vi "Thorlabs-Update Settings.vi"(8 "error in (no error)":errorcluster, 10 "params":variant=variant(cluster{"New LSM Settings":cluster{"Multi Frame Count":dbl, "Trigger Mode":dbl, "Channel Selection":enum32{"A", "B", "AB"}, "Pixel Count":cluster{"Pixels in X":u32, "Pixels in Y":u32}, "Field Size":dbl, "Area Mode":dbl, "Frames":u8, "Averaging":bool, "Alignment":dbl, "Scan Mode":bool, "Gain":cluster{"Gain A":u8, "Gain B":u8}, "Enable PMTs":cluster{"A":bool, "B":bool}, "Voltage Range":cluster{"Range A":u16, "Range B":u16}, "Real Time Averaging":bool, "PFOV":dbl, "MicronsPerPx":dbl}, "index of element":i32} {"New LSM Settings"={"Multi Frame Count"=0.0, "Trigger Mode"=2.0, "Channel Selection"=enum."A", "Pixel Count"={"Pixels in X"=32, "Pixels in Y"=32}, "Field Size"=90.0, "Area Mode"=1.0, "Frames"=2, "Averaging"=FALSE, "Alignment"=0.0, "Scan Mode"=TRUE, "Gain"={"Gain A"=1, "Gain B"=1}, "Enable PMTs"={"A"=TRUE, "B"=TRUE}, "Voltage Range"={"Range A"=10, "Range B"=10}, "Real Time Averaging"=TRUE, "PFOV"=0.0, "MicronsPerPx"=0.0}, "index of element"=13})) -> (0 "error out":errorcluster, 2 "Pause Live Imaging":bool)   [LabVIEW 2020]
uses:
  _Controls/Confocal Controls.ctl
  _Globals/Global Controls.vi
  _Globals/pDataBuffer.vi
  LSM_SDK/ThorConfocal.lvlib
  ECU_SDK/ThorECU.lvlib
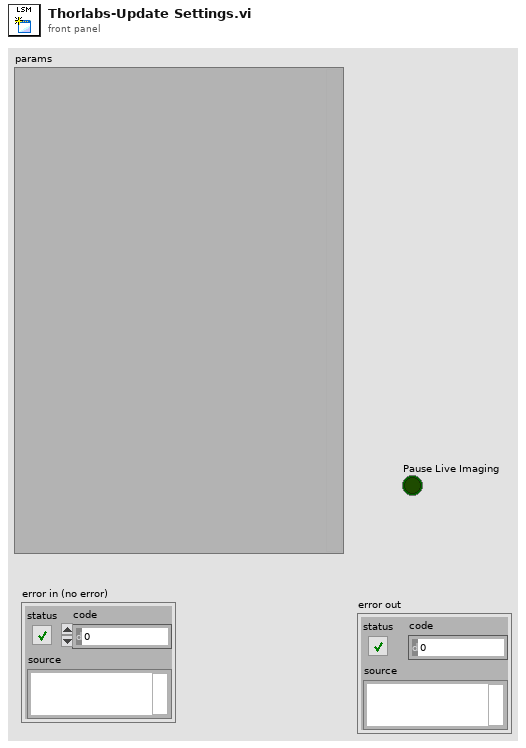
[diagram p1: front panel]
types:
  T1 = typedef "Confocal Controls.ctl" = cluster{"Channel Selection":enum32{"A", "B", "AB"}, "Pixel Count":cluster{"Pixels in X":u32, "Pixels in Y":u32}, "Field Size":dbl, "Frames":u8, "Averaging":bool, "Alignment":dbl, "Scan Mode":bool, "Gain":cluster{"Gain A":u8, "Gain B":u8}, "Enable PMTs":cluster{"A":bool, "B":bool}, "Voltage Range":cluster{"Range A":u16, "Range B":u16}, "Multi Frame Count":dbl, "Trigger Mode":dbl, "Real Time Averaging":bool, "PFOV":dbl, "MicronsPerPx":dbl}
  T2 = cluster{"Newest LSM Settings":T1, "Index of Change":i32}
  T3 = typedef "Tweezertron Ctrl Refs.ctl" = cluster{"LSM Settings":refnum<vi>, "iFlex Control":refnum<vi>, "PIFOC Settings":refnum<vi>, "PinSelector":refnum<vi>, "Manlight Controls":refnum<vi>, "Exp Params":refnum<vi>, "Image Thresholds":refnum<vi>}
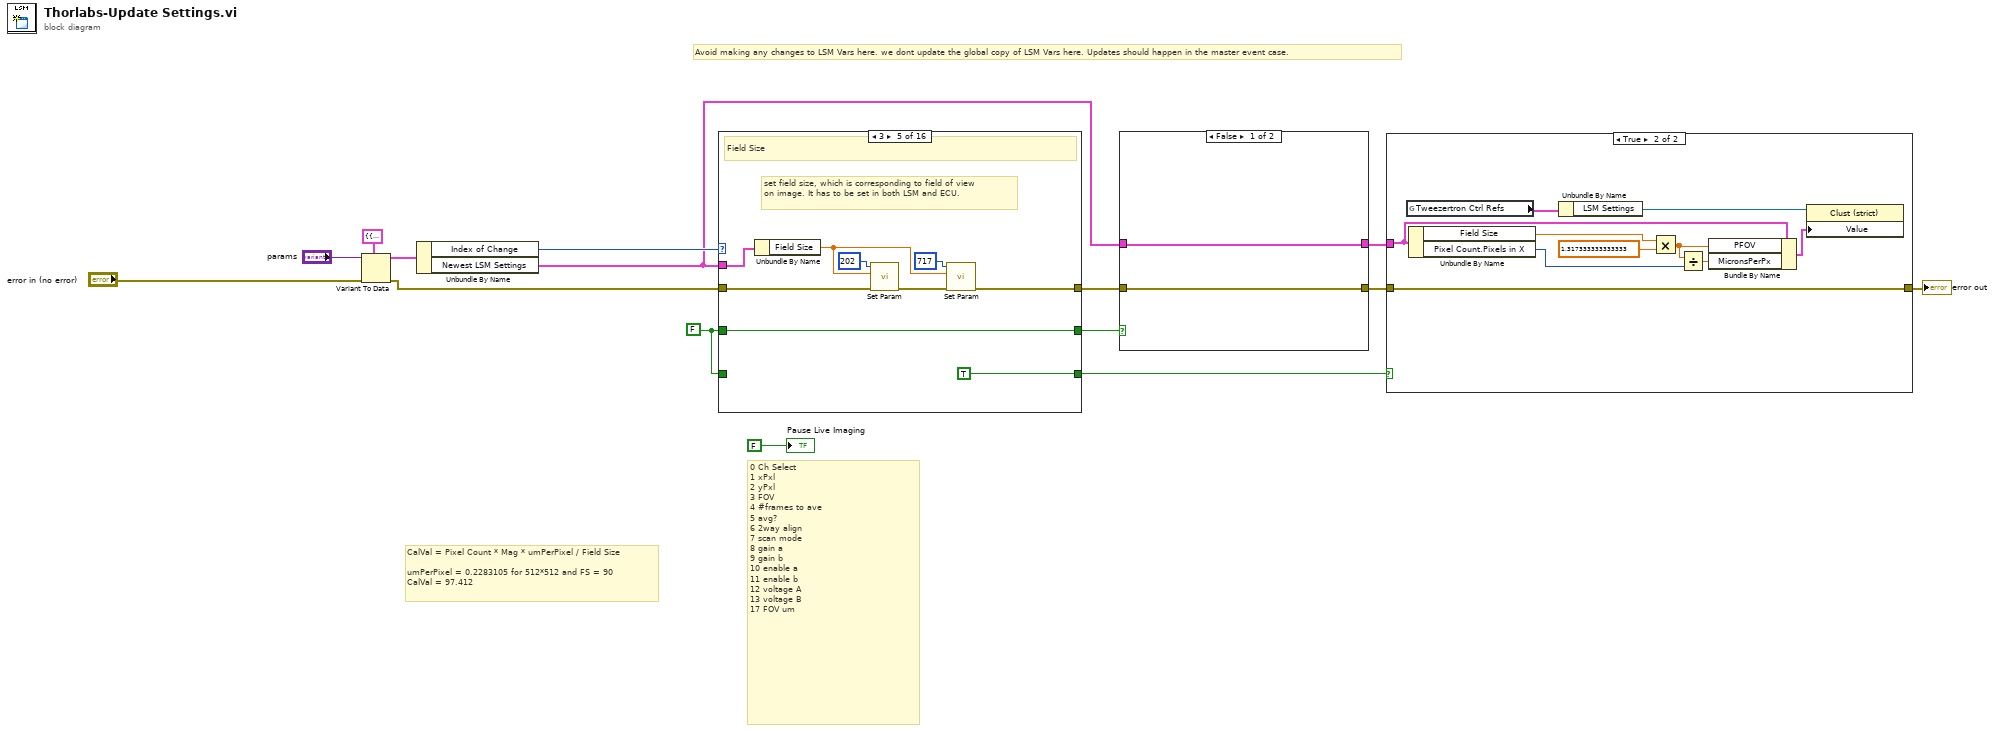
[diagram p0: block diagram]
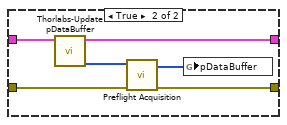
[diagram p3: hidden frame]
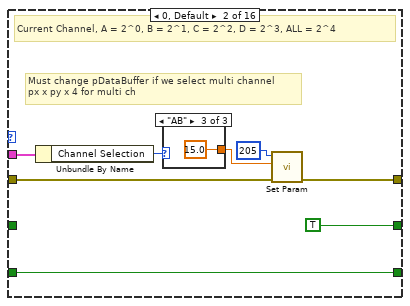
[diagram p5: hidden frame]
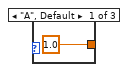
[diagram p6: hidden frame]
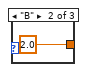
[diagram p7: hidden frame]
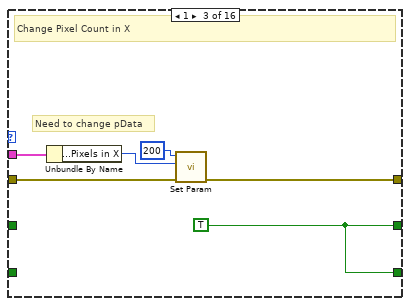
[diagram p8: hidden frame]
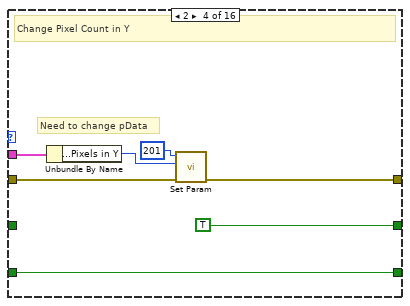
[diagram p9: hidden frame]
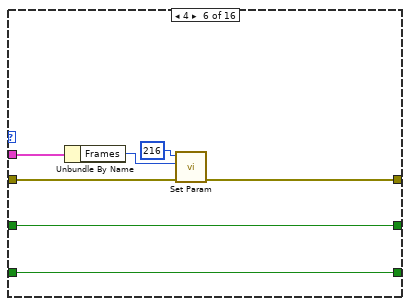
[diagram p10: hidden frame]
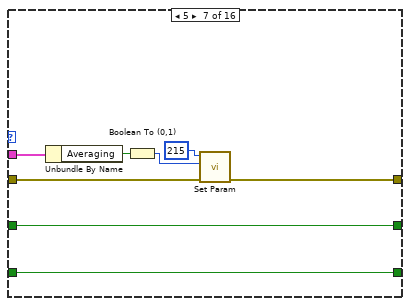
[diagram p11: hidden frame]
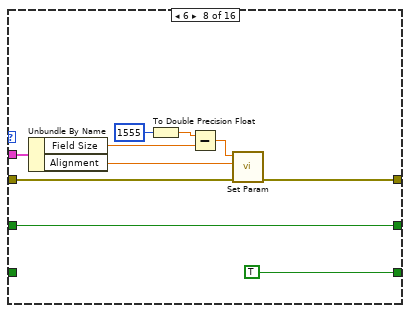
[diagram p12: hidden frame]
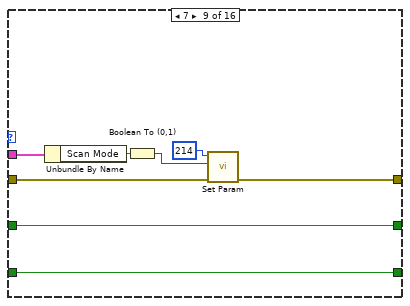
[diagram p13: hidden frame]
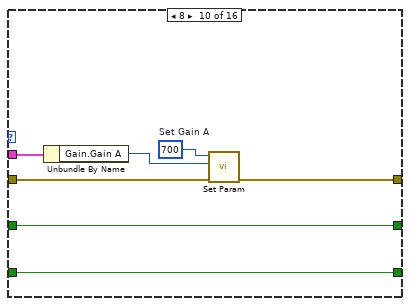
[diagram p14: hidden frame]
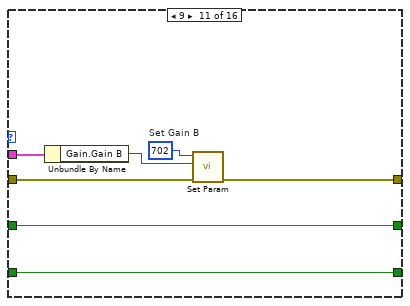
[diagram p15: hidden frame]
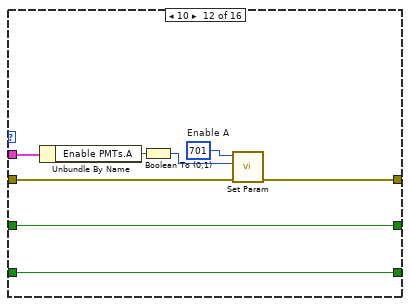
[diagram p16: hidden frame]
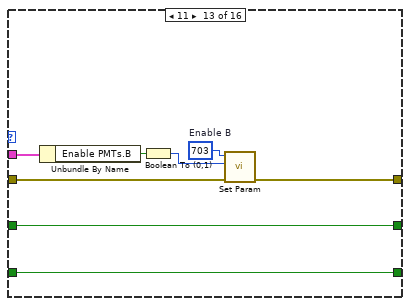
[diagram p17: hidden frame]
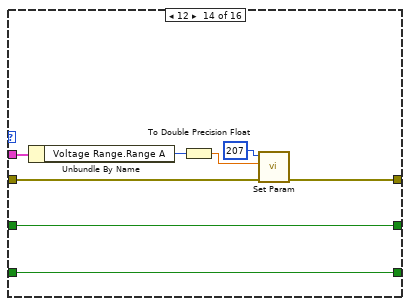
[diagram p18: hidden frame]
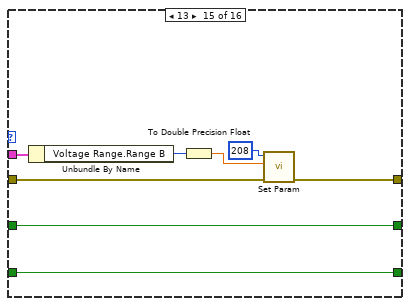
[diagram p19: hidden frame]
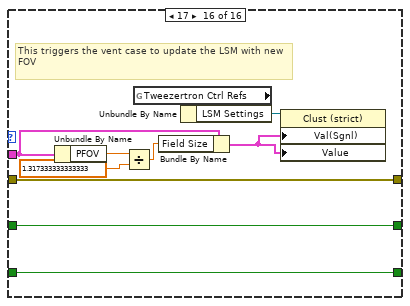
[diagram p20: hidden frame]
diagram:
  w5 = FALSE
  # "Avoid making any changes to LSM Vars here. we dont update the global copy of LSM Vars here. Updates should happen in the master event case."
  # "CalVal = Pixel Count * Mag * umPerPixel / Field Size\n\numPerPixel = 0.2283105 for 512*512 and FS = 90\nCalVal = 97.412"
  # "0 Ch Select \n1 xPxl\n2 yPxl\n3 FOV\n4 #frames to ave\n5 avg?\n6 2way align\n7 scan mode\n8 gain a\n9 gain b\n10 enable a\n11 enable b\n12 voltage A\n13 voltage B\n17 FOV um"
  n1 = Variant To Data(error in="error in (no error)", type=T2 {"Newest LSM Settings"={"Channel Selection"=enum."A", "Pixel Count"={"Pixels in X"=512, "Pixels in Y"=512}, "Field Size"=30.0, "Frames"=0, "Averaging"=FALSE, "Alignment"=0.0, "Scan Mode"=TRUE, "Gain"={"Gain A"=0, "Gain B"=0}, "Enable PMTs"={"A"=FALSE, "B"=FALSE}, "Voltage Range"={"Range A"=10, "Range B"=7}, "Multi Frame Count"=0.0, "Trigger Mode"=2.0, "Real Time Averaging"=TRUE, "PFOV"=0.0, "MicronsPerPx"=0.0}, "Index of Change"=0} ("output cluster"), Variant="params") -> (data=w13:T2, error out=w11:errorcluster)
  n2 = Unbundle By Name(w13) -> ("Index of Change"=w15:i32, "Newest LSM Settings"=w6:T1)
  n3 = case shown="3" w15 {
    tunnel: w6 -> [_ w23 w32 w39 w46 w56 w63 w74 w82 w90 w94 w104 w109 w117 w128 w134]
    tunnel: w11 -> [w18 w25 w35 w42 w51 w58 w66 w76 w84 w88 w96 w106 w111 w122 w129 w133]
    tunnel: [w18 w24 w34 w41 w49 w54 w65 w75 w79 w87 w95 w105 w110 w121 w127 w133] -> w7
    tunnel: [w17 TRUE w30 TRUE w44 w53 w60 w68 w78 w86 w93 w100 w108 w116 w124 w140] -> w8
    tunnel: w5 -> [w17 _ _ _ w44 w53 w60 w68 w78 w86 w93 w100 w108 w116 w124 w140]
    tunnel: w5 -> [w16 w19 _ w36 _ w52 w59 _ w77 w85 w92 w99 w107 w115 w123 w132]
    tunnel: [w16 w19 w30 w36 TRUE w52 w59 TRUE w77 w85 w92 w99 w107 w115 w123 w132] -> w4
    frame -1 {
      # "If nothing changed, do nothing"
    }
    frame 0, Default {
      # "Must change pDataBuffer if we select multi channel\npx x py x 4 for multi ch"
      # "Current Channel, A = 2^0, B = 2^1, C = 2^2, D = 2^3, ALL = 2^4"
      n4 = Unbundle By Name(w23) -> ("Channel Selection"=w22:enum32{"A", "B", "AB"})
      n5 = case shown="\"AB\"" w22 {
        tunnel: [1.0 ("f") 2.0 15.0] -> w21
        frame "A", Default {
        }
        frame "B" {
        }
        frame "AB" {
        }
      }
      n6 = call "Set Param.vi"("error in (no error)"=w25, "param"=w21, "paramID"=205) -> ("error out"=w24:errorcluster)  [unwired: 3 in, 1 out]
    }
    frame 1 {
      w30 = TRUE
      # "Need to change pData"
      # "Change Pixel Count in X"
      n7 = Unbundle By Name(w32) -> ("Pixel Count.Pixels in X"=w31:u32)
      n8 = call "Set Param.vi"("error in (no error)"=w35, "param"=w31, "paramID"=200) -> ("error out"=w34:errorcluster)  [unwired: 3 in, 1 out]
    }
    frame 2 {
      # "Need to change pData"
      # "Change Pixel Count in Y"
      n9 = Unbundle By Name(w39) -> ("Pixel Count.Pixels in Y"=w38:u32)
      n10 = call "Set Param.vi"("error in (no error)"=w42, "param"=w38, "paramID"=201) -> ("error out"=w41:errorcluster)  [unwired: 3 in, 1 out]
    }
    frame 3 {
      # "set field size, which is corresponding to field of view \non image. It has to be set in both LSM and ECU."
      # "Field Size"
      n11 = Unbundle By Name(w46) -> ("Field Size"=w45:dbl)
      n12 = call "Set Param.vi"("error in (no error)"=w51, "param"=w45, "paramID"=202) -> ("error out"=w50:errorcluster)  [unwired: 3 in, 1 out]
      n13 = call "Set Param.vi"("error in (no error)"=w50, "param"=w45, "paramID"=717) -> ("error out"=w49:errorcluster)  [unwired: 7 in, 1 out]
    }
    frame 4 {
      n14 = Unbundle By Name(w56) -> ("Frames"=w55:u8)
      n15 = call "Set Param.vi"("error in (no error)"=w58, "param"=w55, "paramID"=216) -> ("error out"=w54:errorcluster)  [unwired: 3 in, 1 out]
    }
    frame 5 {
      n16 = Unbundle By Name(w63) -> ("Averaging"=w62:bool)
      n17 = Boolean To (0,1)(Boolean=w62) -> (0, 1=w61:i16)
      n18 = call "Set Param.vi"("error in (no error)"=w66, "param"=w61, "paramID"=215) -> ("error out"=w65:errorcluster)  [unwired: 3 in, 1 out]
    }
    frame 6 {
      n19 = Unbundle By Name(w74) -> ("Field Size"=w71:dbl, "Alignment"=w73:dbl)
      n20 = To Double Precision Float(number=1555 ("paramID")) -> (double precision float=w69:dbl)
      n21 = Subtract(x=w69, y=w71) -> (x-y=w70:dbl)
      n22 = call "Set Param.vi"("error in (no error)"=w76, "param"=w73, "paramID"=w70) -> ("error out"=w75:errorcluster)  [unwired: 7 in, 1 out]
    }
    frame 7 {
      n23 = Unbundle By Name(w82) -> ("Scan Mode"=w81:bool)
      n24 = Boolean To (0,1)(Boolean=w81) -> (0, 1=w80:i16)
      n25 = call "Set Param.vi"("error in (no error)"=w84, "param"=w80, "paramID"=214) -> ("error out"=w79:errorcluster)  [unwired: 3 in, 1 out]
    }
    frame 8 {
      w91 = 700  # Set Gain A
      n26 = Unbundle By Name(w90) -> ("Gain.Gain A"=w89:u8)
      n27 = call "Set Param.vi"("error in (no error)"=w88, "param"=w89, "paramID"=w91) -> ("error out"=w87:errorcluster)  [unwired: 7 in, 1 out]
    }
    frame 9 {
      w97 = 702  # Set Gain B
      n28 = Unbundle By Name(w94) -> ("Gain.Gain B"=w98:u8)
      n29 = call "Set Param.vi"("error in (no error)"=w96, "param"=w98, "paramID"=w97) -> ("error out"=w95:errorcluster)  [unwired: 7 in, 1 out]
    }
    frame 10 {
      w102 = 701  # Enable A
      n30 = Unbundle By Name(w104) -> ("Enable PMTs.A"=w103:bool)
      n31 = Boolean To (0,1)(Boolean=w103) -> (0, 1=w101:i16)
      n32 = call "Set Param.vi"("error in (no error)"=w106, "param"=w101, "paramID"=w102) -> ("error out"=w105:errorcluster)  [unwired: 7 in, 1 out]
    }
    frame 11 {
      w112 = 703  # Enable B
      n33 = Unbundle By Name(w109) -> ("Enable PMTs.B"=w113:bool)
      n34 = Boolean To (0,1)(Boolean=w113) -> (0, 1=w114:i16)
      n35 = call "Set Param.vi"("error in (no error)"=w111, "param"=w114, "paramID"=w112) -> ("error out"=w110:errorcluster)  [unwired: 7 in, 1 out]
    }
    frame 12 {
      n36 = Unbundle By Name(w117) -> ("Voltage Range.Range A"=w119:u16)
      n37 = To Double Precision Float(number=w119) -> (double precision float=w118:dbl)
      n38 = call "Set Param.vi"("error in (no error)"=w122, "param"=w118, "paramID"=207) -> ("error out"=w121:errorcluster)  [unwired: 3 in, 1 out]
    }
    frame 13 {
      n39 = Unbundle By Name(w128) -> ("Voltage Range.Range B"=w126:u16)
      n40 = To Double Precision Float(number=w126) -> (double precision float=w125:dbl)
      n41 = call "Set Param.vi"("error in (no error)"=w129, "param"=w125, "paramID"=208) -> ("error out"=w127:errorcluster)  [unwired: 3 in, 1 out]
    }
    frame 17 {
      # "This triggers the vent case to update the LSM with new FOV"
      n42 = Unbundle By Name(w134) -> ("PFOV"=w139:dbl)
      n43 = Divide(x=w139, y=1.317333333333333) -> (x/y=w135:dbl)
      n44 = global read "Global Controls.vi" "Tweezertron Ctrl Refs"() -> (w137:T3)
      n45 = Bundle By Name(cluster=w134, "Field Size"=w135) -> (w131:T1)
      n46 = Unbundle By Name(w137) -> ("LSM Settings"=w136:refnum<vi>)
      n47 = property class="Clust (strict)"(reference=w136, "Val(Sgnl)"=w131, "Value"=w131) -> ()  [unwired: 1 in, 2 out]
    }
  }
  n48 = case shown="False" w8 {
    tunnel: w7 -> [w142 w147]
    tunnel: [w142 w146] -> w2
    tunnel: w6 -> [w141 w144]
    tunnel: [w141 w143] -> w3
    frame False {
    }
    frame True {
      n49 = call "Thorlabs-Update pDataBuffer.vi"("LSM Settings"=w144) -> ("New pDataBuffer"=w145:u16[], "LSM Settings out"=w143:T1)  [unwired: 9 in]
      n50 = call "Preflight Acquisition.vi"("error in (no error)"=w147, "pDataBuffer in"=w145) -> ("error out"=w146:errorcluster, "pDataBuffer out"=w148:u16[])  [unwired: 3 in, 1 out]
      n51 = global write "pDataBuffer.vi" "pDataBuffer"(w148) -> ()
    }
  }
  n52 = case shown="True" w4 {
    tunnel: w3 -> [_ w159]
    tunnel: [w149 w158] -> w1
    tunnel: w2 -> [w149 w158]
    frame False {
    }
    frame True {
      n53 = global read "Global Controls.vi" "Tweezertron Ctrl Refs"() -> (w157:T3)
      n54 = Unbundle By Name(w159) -> ("Field Size"=w154:dbl, "Pixel Count.Pixels in X"=w151:u32)
      n55 = Unbundle By Name(w157) -> ("LSM Settings"=w156:refnum<vi>)
      n56 = Multiply(x=w154, y=1.317333333333333) -> (x*y=w152:dbl)
      n57 = Divide(x=w152, y=w151) -> (x/y=w153:dbl)
      n58 = Bundle By Name(cluster=w159, "PFOV"=w152, "MicronsPerPx"=w153) -> (w155:T1)
      n59 = property class="Clust (strict)"(reference=w156, "Value"=w155) -> ()  [unwired: 1 in, 2 out]
    }
  }
  "error out" <- w1
  "Pause Live Imaging" <- FALSE ("Execution:Suspend On Call")
